vi "main.vi"() -> ()   [LabVIEW 2023]
panel:
  out "Boolean":bool
  in  "Ring 2":u16(ring)
  in  "Ring":u16(ring)
  in  "Game Board":void[][](array[numeric])
  in  "Array":void[][](array[numeric])
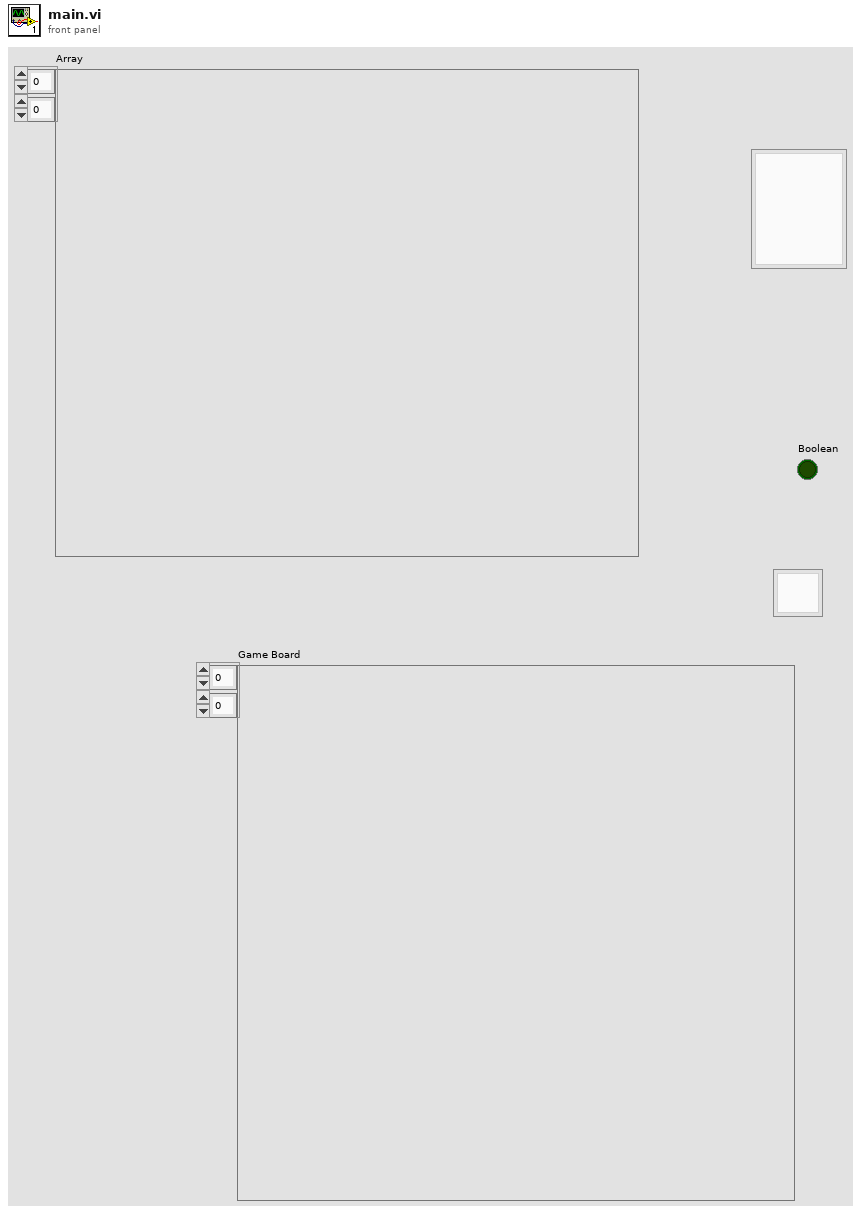
[diagram p1: front panel]
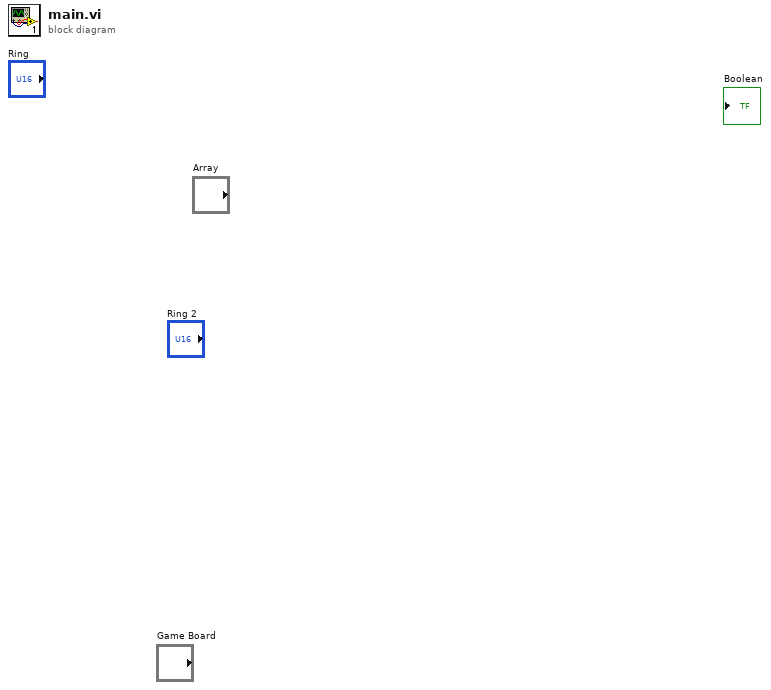
[diagram p0: block diagram]
diagram:
